vi "Get_Client_Status_string.vi"(2 "Client State Cluster":T1={"Client Name"="", "Traverse level State"=enum."Complete", "People to Email"=[], "Next Contact Time"=0.0}, 3 "Client Name":string) -> (0 "Code Value":dbl=14.0 format="%.2f")   [LabVIEW 2020]
uses:
  ADAM Client/Sub VIs/ADAM Controls/Client_State_Cluster.ctl
  ADAM Client/Sub VIs/ADAM Controls/Traverse_Level_State.ctl
  ADAM Client/Sub VIs/ADAM Controls/Remember_value_mode.ctl
  ADAM_Global.vi
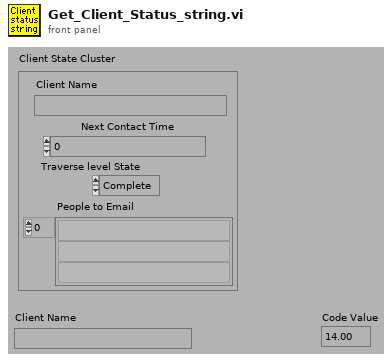
[diagram p1: front panel]
types:
  T1 = typedef "Client_State_Cluster.ctl" = cluster{"Client Name":string, "Traverse level State":T2, "People to Email":string[], "Next Contact Time":dbl}
  T2 = typedef "Traverse_Level_State.ctl" = enum16{"Running", "Complete"}
  T3 = typedef "Remember_value_mode.ctl" = enum16{"Read only", "Read and Write"}
  T4 = cluster{"second":i32, "minute":i32, "hour":i32, "day of month":i32, "month":i32, "year":i32, "day of week":i32, "day of year":i32, "is DST":i32}
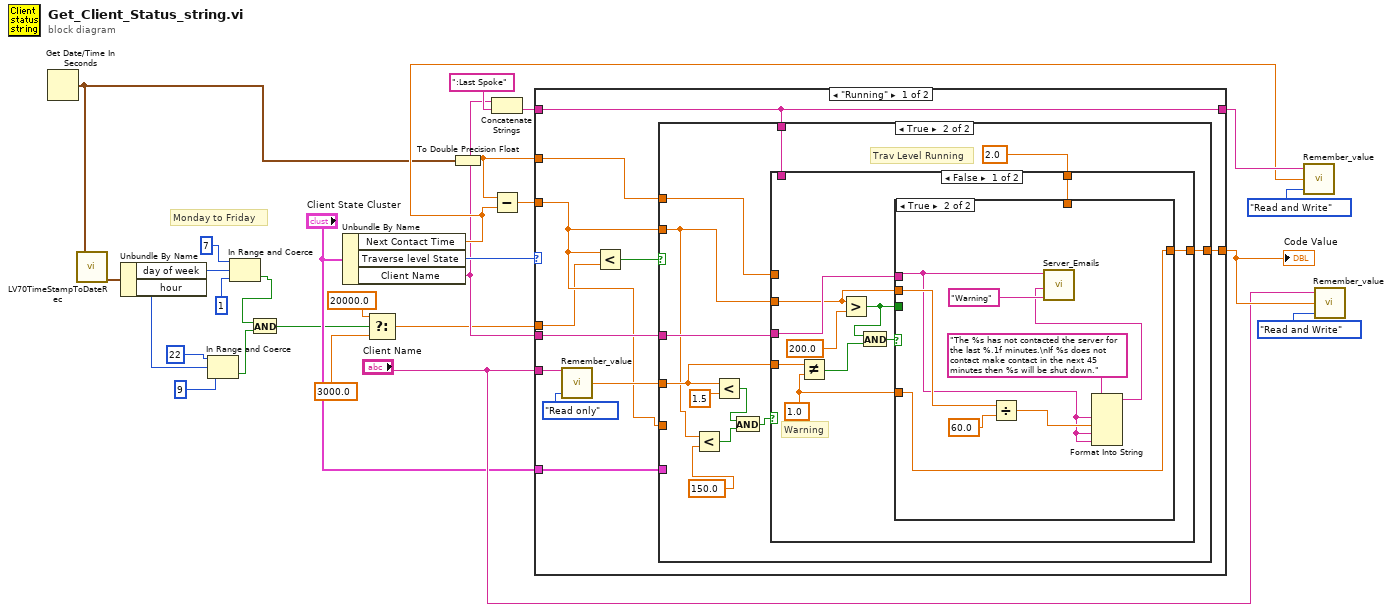
[diagram p0: block diagram]
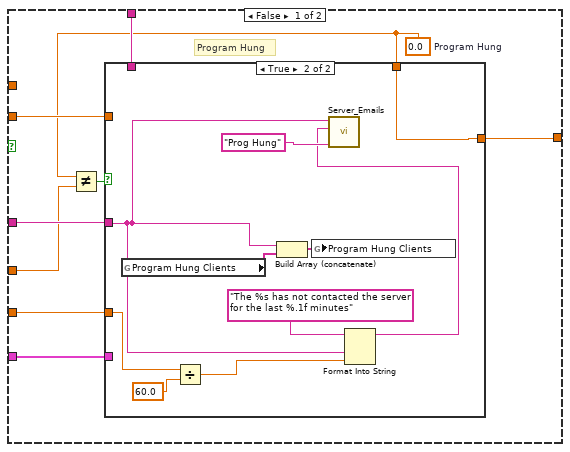
[diagram p2: hidden frame]
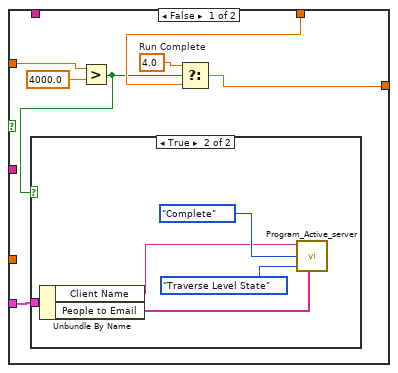
[diagram p3: hidden frame]
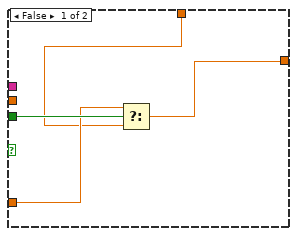
[diagram p5: hidden frame]
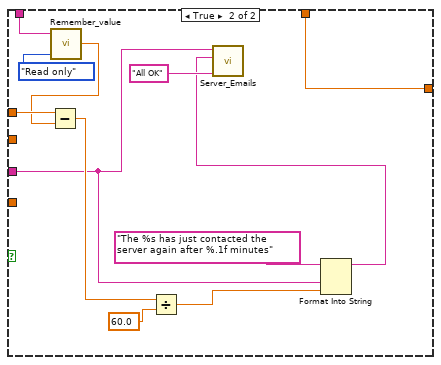
[diagram p6: hidden frame]
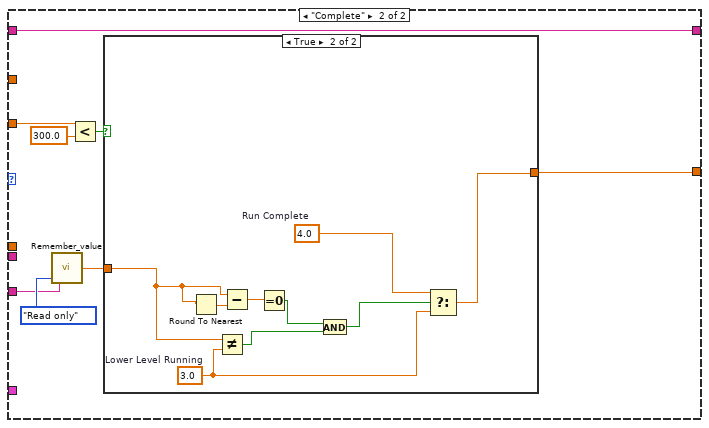
[diagram p7: hidden frame]
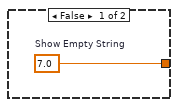
[diagram p8: hidden frame]
diagram:
  # "Monday to Friday"
  n1 = Get Date/Time In Seconds() -> (seconds since 1Jan1904=w5:timestamp)
  n2 = call <vilib>:"LV70TimeStampToDateRec.vi"("time stamp"=w5) -> ("date time rec"=w6:T4)
  n3 = Unbundle By Name(w6) -> ("day of week"=w8:i32, "hour"=w10:i32)
  n4 = In Range and Coerce(upper limit=22, x=w10, lower limit=9) -> (In Range?=w13:bool)  [unwired: 1 out]
  n5 = In Range and Coerce(upper limit=7, x=w8, lower limit=1) -> (In Range?=w14:bool)  [unwired: 1 out]
  n6 = And(x=w14, y=w13) -> (x .and. y?=w4:bool)
  n7 = Unbundle By Name("Client State Cluster") -> ("Next Contact Time"=w18:dbl, "Traverse level State"=w16:T2, "Client Name"=w15:string)
  n8 = Select(t=20000.0 ("y"), s=w4, f=3000.0 ("y")) -> (s? t:f=w1:dbl)
  n9 = To Double Precision Float(number=w5) -> (double precision float=w25:dbl)
  n10 = Concatenate Strings(w15, ":Last Spoke" ("Substring")) -> (w20:string)
  n11 = Subtract(x=w25, y=w18) -> (x-y=w24:dbl)
  n12 = case shown="\"Running\"" w16 {
    tunnel: w25 -> [w31 _]
    tunnel: [w37 w117] -> w26
    tunnel: "Client Name" -> [w34 w119]
    tunnel: w24 -> [w29 w123]
    tunnel: w15 -> [w36 _]
    tunnel: [w32 w116] -> w19
    tunnel: w20 -> [w32 w116]
    tunnel: "Client State Cluster" -> [w30 _]
    tunnel: w1 -> [w28 _]
    frame "Running" {
      n13 = call "Remember_value.vi"("Mode"=Remember_value_mode."Read only", "Ch name"=w34) -> ("Output Value"=w33:dbl)  [unwired: 1 in]
      n14 = Less?(x=w29, y=w28) -> (x < y?=w38:bool)
      n15 = case shown="True" w38 {
        tunnel: [w41 w78] -> w37
        tunnel: w29 -> [w46 _]
        tunnel: w36 -> [w45 w81]
        tunnel: w33 -> [w44 w76]
        tunnel: w32 -> [w43 w80]
        tunnel: w31 -> [_ w79]
        tunnel: w29 -> [w42 w74]
        tunnel: w30 -> [w39 _]
        frame False {
          w40 = 0.0  # Program Hung
          # "Program Hung"
          n16 = Not Equal?(x=w40, y=w44) -> (x != y?=w47:bool)
          n17 = case shown="True" w47 {
            tunnel: w45 -> [_ w60]
            tunnel: w46 -> [_ w63]
            tunnel: w43 -> [_ _]
            tunnel: w42 -> [w54 _]
            tunnel: [w50 w66] -> w41
            tunnel: w40 -> [w52 w66]
            tunnel: w39 -> [w49 _]
            frame False {
              w51 = 4.0  # Run Complete
              n18 = Greater?(x=w54, y=4000.0) -> (0:w48:bool)
              n19 = case shown="True" w48 {
                tunnel: w49 -> [_ w59]
                frame False {
                }
                frame True {
                  n20 = Unbundle By Name(w59) -> ("Client Name"=w55:string, "People to Email"=w58:string[])
                  n21 = call "Program_Active_server.vi"("Client Name"=w55, "Traverse level State"=Traverse_Level_State."Complete", "Mode"=enum16{"Program Active", "Traverse Level State"}."Traverse Level State", "People to Email"=w58) -> ()  [unwired: 2 in, 5 out]
                }
              }
              n22 = Select(t=w51, s=w48, f=w52) -> (s? t:f=w50:dbl)
            }
            frame True {
              n23 = global read "ADAM_Global.vi" "Program Hung Clients"() -> (w62:string[])
              n24 = Divide(x=w63, y=60.0) -> (x/y=w65:dbl)
              n25 = Build Array (concatenate)(w60, w62) -> (w61:string[])
              n26 = global write "ADAM_Global.vi" "Program Hung Clients"(w61) -> ()
              n27 = Format Into String(format string="The %s has not contacted the server for the last %.1f minutes" ("Format String"), w60, w65) -> (resulting string=w67:string)  [unwired: 2 in, 1 out]
              n28 = call "Server_Emails.vi"("Client Name Contains"=w60, "Message"=w67, "Subject"="Prog Hung") -> ()  [unwired: 2 in, 3 out]
            }
          }
        }
        frame True {
          # "Trav Level Running"
          n29 = Less?(x=w74, y=150.0) -> (x < y?=w71:bool)
          n30 = Less?(x=w76, y=1.5) -> (x < y?=w72:bool)
          n31 = And(x=w72, y=w71) -> (x .and. y?=w70:bool)
          n32 = case shown="False" w70 {
            tunnel: w81 -> [w85 w104]
            tunnel: w80 -> [_ w113]
            tunnel: w79 -> [_ w112]
            tunnel: w74 -> [w82 _]
            tunnel: 2.0 ("y") -> [w91 w110]
            tunnel: [w90 w110] -> w78
            tunnel: w76 -> [w88 _]
            frame False {
              w84 = 1.0 ("y")
              # "Warning"
              n33 = Not Equal?(x=w88, y=w84) -> (x != y?=w87:bool)
              n34 = Greater?(x=w82, y=200.0) -> (0:w83:bool)
              n35 = And(x=w83, y=w87) -> (x .and. y?=w86:bool)
              n36 = case shown="True" w86 {
                tunnel: w91 -> [w93 _]
                tunnel: [w92 w102] -> w90
                tunnel: w82 -> [_ w98]
                tunnel: w85 -> [_ w96]
                tunnel: w83 -> [w95 _]
                tunnel: w84 -> [w94 w102]
                frame False {
                  n37 = Select(t=w94, s=w95, f=w93) -> (s? t:f=w92:dbl)
                }
                frame True {
                  n38 = Divide(x=w98, y=60.0) -> (x/y=w100:dbl)
                  n39 = Format Into String(format string="The %s has not contacted the server for the last %.1f minutes.\nIf %s does not contact make contact in the next 45 minutes then %s will be shut down." ("Format String"), w96, w100, w96, w96) -> (resulting string=w97:string)  [unwired: 2 in, 1 out]
                  n40 = call "Server_Emails.vi"("Client Name Contains"=w96, "Message"=w97, "Subject"="Warning") -> ()  [unwired: 2 in, 3 out]
                }
              }
            }
            frame True {
              n41 = call "Remember_value.vi"("Mode"=Remember_value_mode."Read only", "Ch name"=w113) -> ("Output Value"=w111:dbl)  [unwired: 1 in]
              n42 = Subtract(x=w112, y=w111) -> (x-y=w106:dbl)
              n43 = Divide(x=w106, y=60.0) -> (x/y=w108:dbl)
              n44 = Format Into String(format string="The %s has just contacted the server again after %.1f minutes" ("Format String"), w104, w108) -> (resulting string=w105:string)  [unwired: 2 in, 1 out]
              n45 = call "Server_Emails.vi"("Client Name Contains"=w104, "Message"=w105, "Subject"="All OK") -> ()  [unwired: 2 in, 3 out]
            }
          }
        }
      }
    }
    frame "Complete" {
      n46 = call "Remember_value.vi"("Mode"=Remember_value_mode."Read only", "Ch name"=w119) -> ("Output Value"=w118:dbl)  [unwired: 1 in]
      n47 = Less?(x=w123, y=300.0) -> (x < y?=w121:bool)
      n48 = case shown="True" w121 {
        tunnel: w118 -> [_ w129]
        tunnel: [w124 w130] -> w117
        frame False {
          w124 = 7.0  # Show Empty String
        }
        frame True {
          w131 = 4.0  # Run Complete
          w128 = 3.0  # Lower Level Running
          n49 = Round To Nearest(number=w129) -> (nearest integer value=w133:dbl)
          n50 = Not Equal?(x=w129, y=w128) -> (x != y?=w127:bool)
          n51 = Subtract(x=w129, y=w133) -> (x-y=w132:dbl)
          n52 = Equal To 0?(x=w132) -> (x = 0?=w126:bool)
          n53 = And(x=w126, y=w127) -> (x .and. y?=w125:bool)
          n54 = Select(t=w131, s=w125, f=w128) -> (s? t:f=w130:dbl)
        }
      }
    }
  }
  "Code Value" <- w26
  n55 = call "Remember_value.vi"("Mode"=Remember_value_mode."Read and Write", "Input Value"=w18, "Ch name"=w19) -> ()  [unwired: 1 out]
  n56 = call "Remember_value.vi"("Mode"=Remember_value_mode."Read and Write", "Input Value"=w26, "Ch name"="Client Name") -> ()  [unwired: 1 out]
